vi "Get Actuator.vi"(11 "Model in":refnum<class "Model.lvclass">) -> (2 "Actuator.lvclass":refnum<class "Actuator.lvclass">, 3 "Model out":refnum<class "Model.lvclass">)   [LabVIEW 2015, in "Model.lvclass"]
uses:
  Model.lvclass
  Actuator/Actuator/Actuator.lvclass
  Model.lvclass/Model.ctl
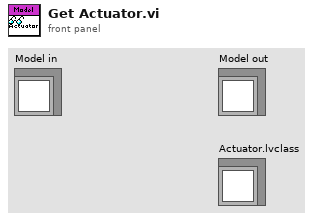
[diagram p1: front panel]
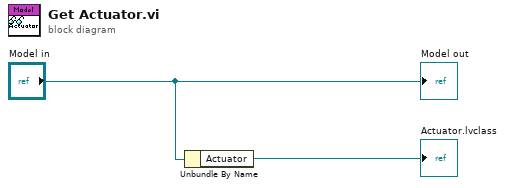
[diagram p0: block diagram]
diagram:
  n1 = Unbundle By Name("Model in") -> ("Actuator"=→"Actuator.lvclass":refnum<class "Actuator.lvclass">)
  "Model out" <- "Model in"
